vi "机械臂-labview控制仿真.vi"() -> ()   [LabVIEW 2012]
doc: "主要是学习如何用LabView控制三维模型，现在只是手动控制，以后有时间把它完善为可以按程序运行的软件，让它自动计算出运行路径（三维），把机械臂相对于直角坐标机床的优势充分发掘出来，现在比较粗糟，见笑了!注：机械臂的模型是从互联网上下载的，我只是把它转换为WRL文件而已，我非常感谢原作者！感谢NI公司开发的LabView软件，让我们身在偏远地方的工程师也可以用仿真的方式学习。我也把这个软件发到互联网上供大家学习，有什么问题可以跟我联系。罗清 电话：13548205451 QQ：564200811"
uses:
  <vilib>/Utility/miscctls.llb/LVRGBAColorTypeDef.ctl
  <vilib>/picture/3D Picture Control/NI_3D Picture Control.lvlib
panel:
  in  "刀具转动":bool=TRUE
  in  "爪头旋转":sgl(knob) scale=0.0..6.28
  in  "关节1旋转":sgl(knob) scale=-0.785..3.925
  in  "小臂旋转":sgl(knob) scale=0.0..6.28
  in  "爪头座旋转":sgl(knob) scale=-1.57..1.57
  in  "背景色":T1={"Red"=0.7, "Green"=0.7, "Blue"=0.7, "Alpha"=0.0}
  in  "关节2旋转":sgl(knob) scale=0.0..6.28
  in  "大臂旋转":sgl(knob) scale=-1.57..1.57
  in  "上下移动":dbl(slide)=-1.0
  in  "机械臂缩放":sgl(knob)=2.0 scale=0.0..4.0
  in  "停止":bool
  out "六自由度机械臂":refnum<vi>(3d-picture)
  # "运行控制"
  # "基本设置"
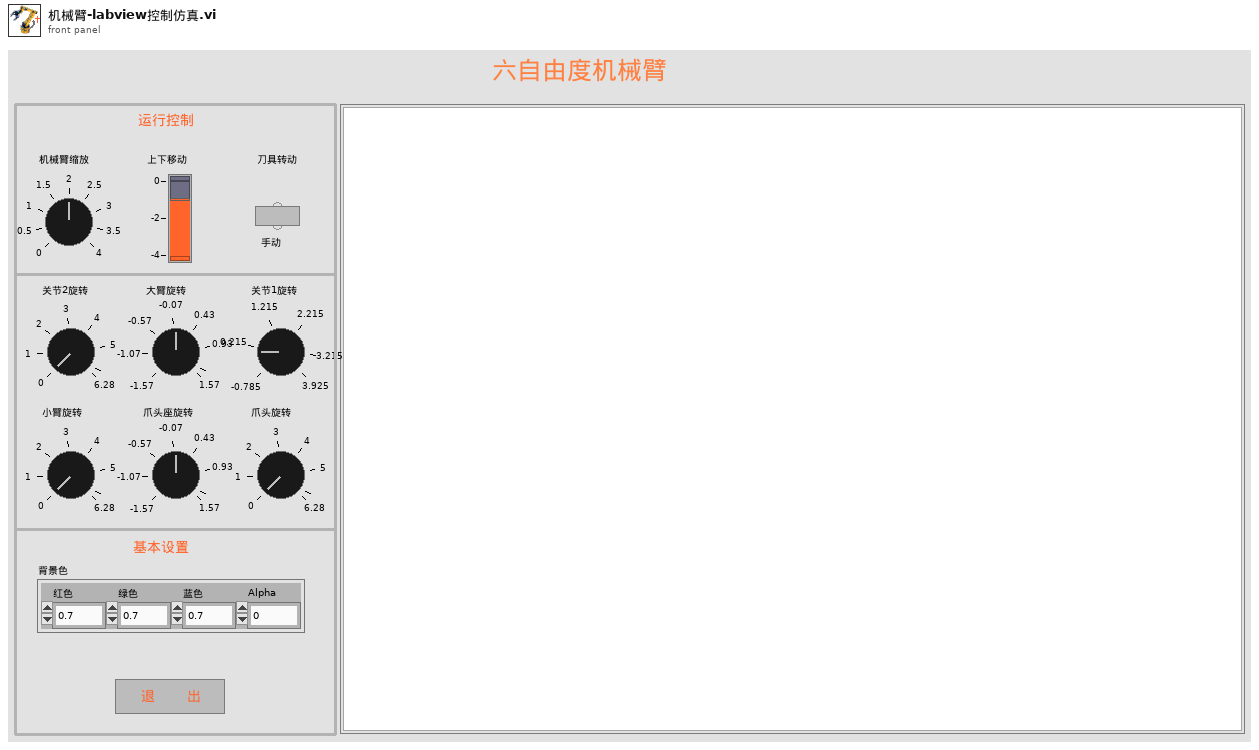
[diagram p1: front panel]
types:
  T1 = typedef "LVRGBAColorTypeDef.ctl" = cluster{"Red":sgl, "Green":sgl, "Blue":sgl, "Alpha":sgl}
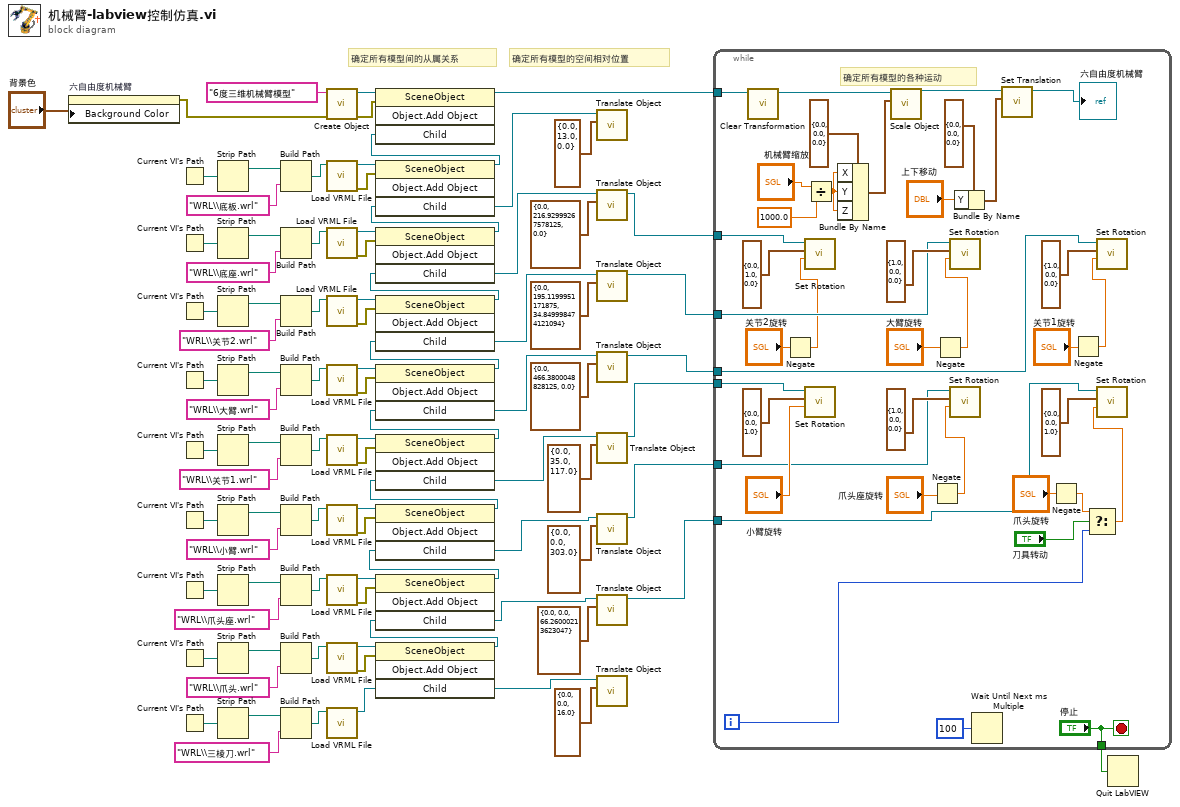
[diagram p0: block diagram]
diagram:
  # "确定所有模型的空间相对位置"
  # "确定所有模型间的从属关系"
  n1 = property on="六自由度机械臂" class="SceneGraphDisp (严格)"("Background Color"="背景色") -> (error out=w2:errorcluster)  [unwired: 2 in, 1 out]
  n2 = Current VI's Path() -> (path=w86:path)
  n3 = Current VI's Path() -> (path=w82:path)
  n4 = Current VI's Path() -> (path=w78:path)
  n5 = Current VI's Path() -> (path=w75:path)
  n6 = Current VI's Path() -> (path=w72:path)
  n7 = Current VI's Path() -> (path=w69:path)
  n8 = Current VI's Path() -> (path=w66:path)
  n9 = Current VI's Path() -> (path=w63:path)
  n10 = Current VI's Path() -> (path=w60:path)
  n11 = Strip Path(path=w86) -> (stripped path=w84:path)  [unwired: 1 out]
  n12 = Strip Path(path=w82) -> (stripped path=w80:path)  [unwired: 1 out]
  n13 = Strip Path(path=w78) -> (stripped path=w76:path)  [unwired: 1 out]
  n14 = Strip Path(path=w75) -> (stripped path=w73:path)  [unwired: 1 out]
  n15 = Strip Path(path=w72) -> (stripped path=w70:path)  [unwired: 1 out]
  n16 = Strip Path(path=w69) -> (stripped path=w67:path)  [unwired: 1 out]
  n17 = Strip Path(path=w66) -> (stripped path=w64:path)  [unwired: 1 out]
  n18 = Strip Path(path=w63) -> (stripped path=w61:path)  [unwired: 1 out]
  n19 = Strip Path(path=w60) -> (stripped path=w58:path)  [unwired: 1 out]
  n20 = Build Path(base path=w84, name or relative path="WRL\\底板.wrl" ("名称或相对路径")) -> (appended path=w83:path)
  n21 = Build Path(base path=w80, name or relative path="WRL\\底座.wrl" ("名称或相对路径")) -> (appended path=w79:path)
  n22 = Build Path(base path=w76, name or relative path="WRL\\关节2.wrl" ("名称或相对路径")) -> (appended path=w57:path)
  n23 = Build Path(base path=w73, name or relative path="WRL\\大臂.wrl" ("名称或相对路径")) -> (appended path=w56:path)
  n24 = Build Path(base path=w70, name or relative path="WRL\\关节1.wrl" ("名称或相对路径")) -> (appended path=w55:path)
  n25 = Build Path(base path=w67, name or relative path="WRL\\小臂.wrl" ("名称或相对路径")) -> (appended path=w54:path)
  n26 = Build Path(base path=w64, name or relative path="WRL\\爪头座.wrl" ("名称或相对路径")) -> (appended path=w53:path)
  n27 = Build Path(base path=w61, name or relative path="WRL\\爪头.wrl" ("名称或相对路径")) -> (appended path=w52:path)
  n28 = Build Path(base path=w58, name or relative path="WRL\\三棱刀.wrl" ("名称或相对路径")) -> (appended path=w51:path)
  n29 = call <vilib>:"Create Object.vi"("error in (no error)"=w2, "Name"="6度三维机械臂模型") -> ("error out"=w88:errorcluster, "Scene:New Object"=w89:refnum<vi>)  [unwired: 8 in]
  n30 = call <vilib>:"Load VRML File.vi"("Path"=w83) -> ("error out"=w29:errorcluster, "Scene:Read Scene File"=w31:refnum<vi>)  [unwired: 9 in]
  n31 = call <vilib>:"Load VRML File.vi"("Path"=w79) -> ("error out"=w38:errorcluster, "Scene:Read Scene File"=w87:refnum<vi>)  [unwired: 9 in]
  n32 = call <vilib>:"Load VRML File.vi"("Path"=w57) -> ("error out"=w39:errorcluster, "Scene:Read Scene File"=w50:refnum<vi>)  [unwired: 9 in]
  n33 = call <vilib>:"Load VRML File.vi"("Path"=w56) -> ("error out"=w40:errorcluster, "Scene:Read Scene File"=w49:refnum<vi>)  [unwired: 9 in]
  n34 = call <vilib>:"Load VRML File.vi"("Path"=w55) -> ("error out"=w41:errorcluster, "Scene:Read Scene File"=w48:refnum<vi>)  [unwired: 9 in]
  n35 = call <vilib>:"Load VRML File.vi"("Path"=w54) -> ("error out"=w42:errorcluster, "Scene:Read Scene File"=w47:refnum<vi>)  [unwired: 9 in]
  n36 = call <vilib>:"Load VRML File.vi"("Path"=w53) -> ("error out"=w45:errorcluster, "Scene:Read Scene File"=w46:refnum<vi>)  [unwired: 9 in]
  n37 = call <vilib>:"Load VRML File.vi"("Path"=w52) -> ("error out"=w43:errorcluster, "Scene:Read Scene File"=w44:refnum<vi>)  [unwired: 9 in]
  n38 = call <vilib>:"Load VRML File.vi"("Path"=w51) -> ("Scene:Read Scene File"=w28:refnum<vi>)  [unwired: 9 in, 1 out]
  n39 = invoke class="SceneObject" method="Object.Add Object"(reference=w44, error in=w43, "Child"=w28) -> (reference out=w32:refnum<vi>, "Child"=w18:refnum<vi>)  [unwired: 1 in, 2 out]
  n40 = invoke class="SceneObject" method="Object.Add Object"(reference=w46, error in=w45, "Child"=w32) -> (reference out=w33:refnum<vi>, "Child"=w10:refnum<vi>)  [unwired: 1 in, 2 out]
  n41 = invoke class="SceneObject" method="Object.Add Object"(reference=w47, error in=w42, "Child"=w33) -> (reference out=w34:refnum<vi>, "Child"=w19:refnum<vi>)  [unwired: 1 in, 2 out]
  n42 = invoke class="SceneObject" method="Object.Add Object"(reference=w48, error in=w41, "Child"=w34) -> (reference out=w35:refnum<vi>, "Child"=w21:refnum<vi>)  [unwired: 1 in, 2 out]
  n43 = invoke class="SceneObject" method="Object.Add Object"(reference=w49, error in=w40, "Child"=w35) -> (reference out=w36:refnum<vi>, "Child"=w23:refnum<vi>)  [unwired: 1 in, 2 out]
  n44 = invoke class="SceneObject" method="Object.Add Object"(reference=w50, error in=w39, "Child"=w36) -> (reference out=w37:refnum<vi>, "Child"=w25:refnum<vi>)  [unwired: 1 in, 2 out]
  n45 = invoke class="SceneObject" method="Object.Add Object"(reference=w87, error in=w38, "Child"=w37) -> (reference out=w27:refnum<vi>, "Child"=w11:refnum<vi>)  [unwired: 1 in, 2 out]
  n46 = invoke class="SceneObject" method="Object.Add Object"(reference=w31, error in=w29, "Child"=w27) -> (reference out=w30:refnum<vi>, "Child"=w12:refnum<vi>)  [unwired: 1 in, 2 out]
  n47 = invoke class="SceneObject" method="Object.Add Object"(reference=w89, error in=w88, "Child"=w30) -> (reference out=w13:refnum<vi>)  [unwired: 1 in, 3 out]
  n48 = call <vilib>:"Translate Object.vi"("Translation"=cluster{"X":sgl, "Y":sgl, "Z":sgl} {"X"=0.0, "Y"=13.0, "Z"=0.0}, "Scene.Object In"=w12) -> ()  [unwired: 8 in, 2 out]
  n49 = call <vilib>:"Translate Object.vi"("Translation"=cluster{"X":sgl, "Y":sgl, "Z":sgl} {"X"=0.0, "Y"=216.93, "Z"=0.0}, "Scene.Object In"=w11) -> ("Scene.Object Out"=w9:refnum<vi>)  [unwired: 8 in, 1 out]
  n50 = call <vilib>:"Translate Object.vi"("Translation"=cluster{"X":sgl, "Y":sgl, "Z":sgl} {"X"=0.0, "Y"=195.12, "Z"=34.85}, "Scene.Object In"=w25) -> ("Scene.Object Out"=w8:refnum<vi>)  [unwired: 8 in, 1 out]
  n51 = call <vilib>:"Translate Object.vi"("Translation"=cluster{"X":sgl, "Y":sgl, "Z":sgl} {"X"=0.0, "Y"=466.38, "Z"=0.0}, "Scene.Object In"=w23) -> ("Scene.Object Out"=w7:refnum<vi>)  [unwired: 8 in, 1 out]
  n52 = call <vilib>:"Translate Object.vi"("Translation"=cluster{"X":sgl, "Y":sgl, "Z":sgl} {"X"=0.0, "Y"=35.0, "Z"=117.0}, "Scene.Object In"=w21) -> ("Scene.Object Out"=w6:refnum<vi>)  [unwired: 8 in, 1 out]
  n53 = call <vilib>:"Translate Object.vi"("Translation"=cluster{"X":sgl, "Y":sgl, "Z":sgl} {"X"=0.0, "Y"=0.0, "Z"=303.0}, "Scene.Object In"=w19) -> ("Scene.Object Out"=w5:refnum<vi>)  [unwired: 8 in, 1 out]
  n54 = call <vilib>:"Translate Object.vi"("Translation"=cluster{"X":sgl, "Y":sgl, "Z":sgl} {"X"=0.0, "Y"=0.0, "Z"=66.26}, "Scene.Object In"=w10) -> ("Scene.Object Out"=w4:refnum<vi>)  [unwired: 8 in, 1 out]
  n55 = call <vilib>:"Translate Object.vi"("Translation"=cluster{"X":sgl, "Y":sgl, "Z":sgl} {"X"=0.0, "Y"=0.0, "Z"=16.0}, "Scene.Object In"=w18) -> ()  [unwired: 8 in, 2 out]
  n56 = while {
    tunnel: w13 -> [w117]
    tunnel: w9 -> [w111]
    tunnel: w8 -> [w110]
    tunnel: w7 -> [w109]
    tunnel: w6 -> [w108]
    tunnel: w5 -> [w107]
    tunnel: w4 -> [w106]
    tunnel: ["停止"] -> w1
    i -> [w94]
    stop <- "停止" stop-if-true
    # "确定所有模型的各种运动"
    n57 = call <vilib>:"Clear Transformation.vi"("Object Refnum In"=w117) -> ("Object Refnum Out"=w130:refnum<vi>)  [unwired: 9 in, 1 out]
    n58 = Negate(x="关节2旋转") -> (-x=w97:sgl)
    n59 = call <vilib>:"Set Rotation.vi"("Angle"=w97, "Axis"=cluster{"X":sgl, "Y":sgl, "Z":sgl} {"X"=0.0, "Y"=1.0, "Z"=0.0}, "Scene Object"=w111) -> ()  [unwired: 7 in, 2 out]
    n60 = call <vilib>:"Set Rotation.vi"("Angle"="小臂旋转", "Axis"=cluster{"X":sgl, "Y":sgl, "Z":sgl} {"X"=0.0, "Y"=0.0, "Z"=1.0}, "Scene Object"=w108) -> ()  [unwired: 7 in, 2 out]
    n61 = Divide(x="机械臂缩放", y=1000.0) -> (x/y=w123:dbl)
    n62 = Bundle By Name(cluster=cluster{"X":sgl, "Y":sgl, "Z":sgl} {"X"=0.0, "Y"=0.0, "Z"=0.0} ("Scale"), "X"=w123, "Y"=w123, "Z"=w123) -> (w126:cluster{"X":sgl, "Y":sgl, "Z":sgl})
    n63 = call <vilib>:"Scale Object.vi"("Scale"=w126, "Scene.Object In"=w130) -> ("Scene.Object Out"=w121:refnum<vi>)  [unwired: 8 in, 1 out]
    n64 = Negate(x="爪头座旋转") -> (-x=w102:sgl)
    n65 = Negate(x="大臂旋转") -> (-x=w104:sgl)
    n66 = call <vilib>:"Set Rotation.vi"("Angle"=w104, "Axis"=cluster{"X":sgl, "Y":sgl, "Z":sgl} {"X"=1.0, "Y"=0.0, "Z"=0.0}, "Scene Object"=w110) -> ()  [unwired: 7 in, 2 out]
    n67 = call <vilib>:"Set Rotation.vi"("Angle"=w102, "Axis"=cluster{"X":sgl, "Y":sgl, "Z":sgl} {"X"=1.0, "Y"=0.0, "Z"=0.0}, "Scene Object"=w107) -> ()  [unwired: 7 in, 2 out]
    n68 = Bundle By Name(cluster=cluster{"X":sgl, "Y":sgl, "Z":sgl} {"X"=0.0, "Y"=0.0, "Z"=0.0} ("Translation"), "Y"="上下移动") -> (w118:cluster{"X":sgl, "Y":sgl, "Z":sgl})
    n69 = Wait Until Next ms Multiple(millisecond multiple=u32 100 ("毫秒倍数")) -> ()  [unwired: 1 out]
    n70 = call <vilib>:"Set Translation.vi"("Translation"=w118, "Scene Object"=w121) -> ("Translated Object"=→"六自由度机械臂":refnum<vi>)  [unwired: 8 in, 1 out]
    n71 = Negate(x="爪头旋转") -> (-x=w96:sgl)
    n72 = Negate(x="关节1旋转") -> (-x=w99:sgl)
    n73 = Select(t=w96, s="刀具转动", f=w94) -> (s? t:f=w93:sgl)
    n74 = call <vilib>:"Set Rotation.vi"("Angle"=w99, "Axis"=cluster{"X":sgl, "Y":sgl, "Z":sgl} {"X"=1.0, "Y"=0.0, "Z"=0.0}, "Scene Object"=w109) -> ()  [unwired: 7 in, 2 out]
    n75 = call <vilib>:"Set Rotation.vi"("Angle"=w93, "Axis"=cluster{"X":sgl, "Y":sgl, "Z":sgl} {"X"=0.0, "Y"=0.0, "Z"=1.0}, "Scene Object"=w106) -> ()  [unwired: 7 in, 2 out]
  }
  n76 = Quit LabVIEW(quit? (T)=w1) -> ()
